vi "playing with digital WF.vi"() -> ()   [LabVIEW 2013]
uses:
  <vilib>/Waveform/DTblOps.llb/DTbl Compress Digital.vi
  <vilib>/Waveform/DTblOps.llb/DTbl Digital Size.vi
panel:
  out "number of signals 2":i32=4
  out "number of samples 2":i32=7
  out "number of signals":i32=4
  out "number of samples":i32=7
  in  "Digital Data":digitaldata={"transitions"=[], "data"=[[0, 0, 0, 0], [0, 1, 0, 0], [0, 1, 0, 0], [0, 0, 1, 0], [0, 0, 1, 0], [0, 0, 1, 0], [0, 0, 0, 0]]}
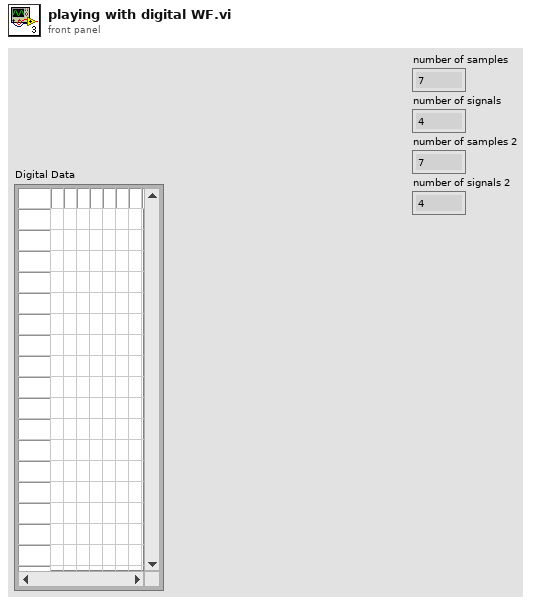
[diagram p1: front panel]
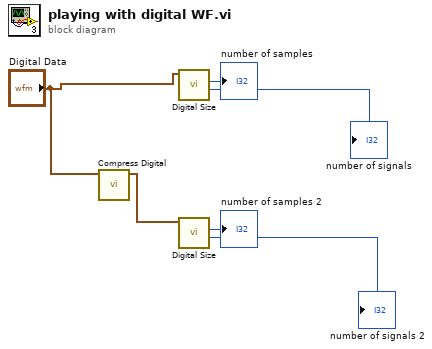
[diagram p0: block diagram]
diagram:
  n1 = call-poly <vilib>:"Compress Digital.vi"("uncompressed digital data"="Digital Data") -> ("compressed digital data"=w3:digitaldata)  [unwired: 9 in, 1 out]
  n2 = call-poly <vilib>:"Digital Size.vi"("digital data in"="Digital Data") -> ("number of signals"=→"number of signals":i32, "number of samples"=→"number of samples":i32)  [unwired: 7 in, 2 out]
  n3 = call-poly <vilib>:"Digital Size.vi"("digital data in"=w3) -> ("number of signals"=→"number of signals 2":i32, "number of samples"=→"number of samples 2":i32)  [unwired: 7 in, 2 out]
